vi "add sensor.vi"(8 "error in (no error)":errorcluster) -> (0 "error out":errorcluster, 1 "new sensor output":string, 3 "Enum":enum16{"OK", "Cancel"}(ring))   [LabVIEW 2023]
panel:
  in  "Cancel":bool
  in  "OK":bool
  in  "new sensor":string
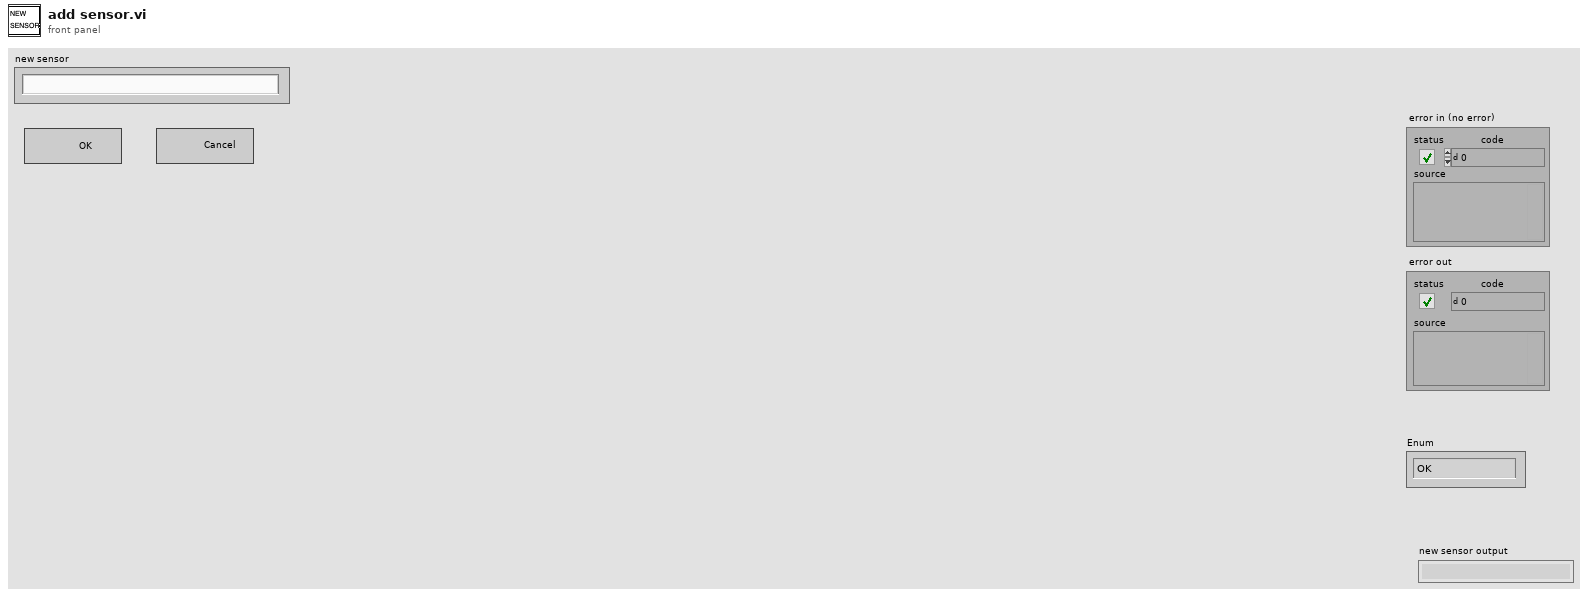
[diagram p1: front panel]
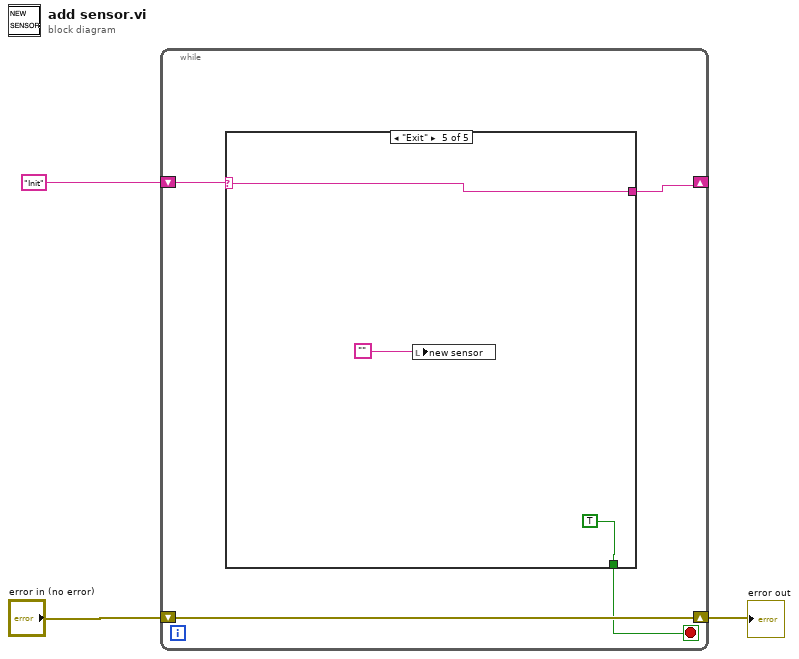
[diagram p0: block diagram]
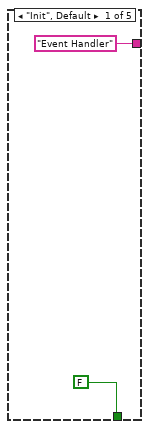
[diagram p2: hidden frame]
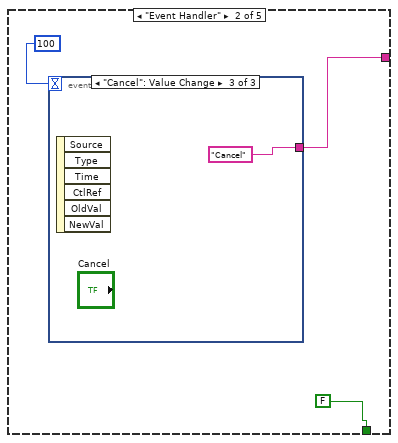
[diagram p3: hidden frame]
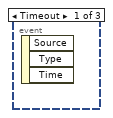
[diagram p4: hidden frame]
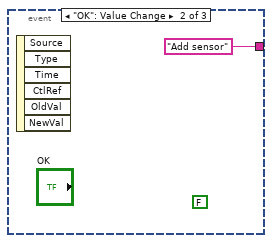
[diagram p5: hidden frame]
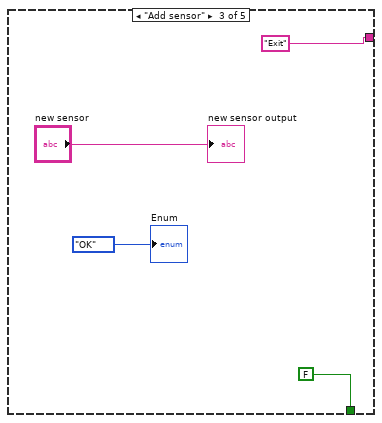
[diagram p6: hidden frame]
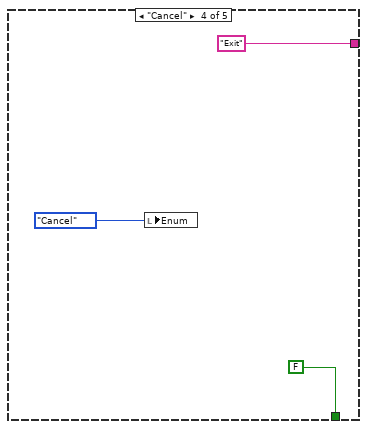
[diagram p7: hidden frame]
diagram:
  n1 = while {
    shift-right: [w6] -> _
    shift-left: "Init" -> [w7]
    shift-right: [w5] -> w1
    shift-left: "error in (no error)" -> [w5]
    stop <- w4 stop-if-true
    n2 = case shown="\"Exit\"" w7 {
      selector: w7 -> [_ _ _ _ w23]
      tunnel: ["Event Handler" w11 "Exit" "Exit" w23] -> w6
      tunnel: [FALSE FALSE FALSE FALSE TRUE] -> w4
      frame "Init", Default {
      }
      frame "Event Handler" {
        n3 = event shown="[2] \"Cancel\": Value Change" {
          selector: _ -> [_ _ _]
          dyn-events: _ -> [_ _ _]
          timeout: 100 -> [_ _ _]
          tunnel: [_ "Add sensor" "Cancel"] -> w11
          event Timeout {
            n4 = event-data() -> ()  [unwired: 1 in, 3 out]
          }
          event "OK": Value Change {
            (unwired) FALSE
            n5 = event-data() -> ()  [unwired: 1 in, 6 out]
          }
          event "Cancel": Value Change {
            n6 = event-data() -> ()  [unwired: 1 in, 6 out]
          }
        }
      }
      frame "Add sensor" {
        "new sensor output" <- "new sensor"
        "Enum" <- enum16{"OK", "Cancel"}."OK" ("Enum")
      }
      frame "Cancel" {
        n7 = local write "Enum"(enum16{"OK", "Cancel"}."Cancel" ("Enum")) -> ()
      }
      frame "Exit" {
        n8 = local write "new sensor"("") -> ()
      }
    }
  }
  "error out" <- w1
